vi "Filter StartRun Msg.vi"(10 "Current List":string, 11 "New RT Events":string) -> (3 "New List":string)   [LabVIEW 2015]
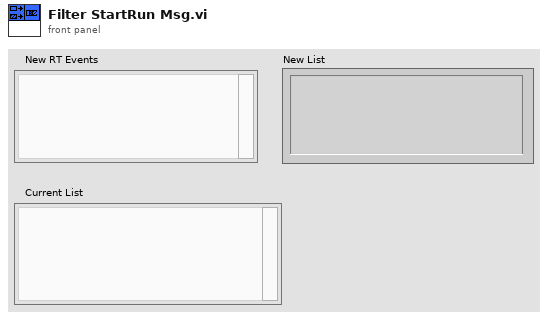
[diagram p1: front panel]
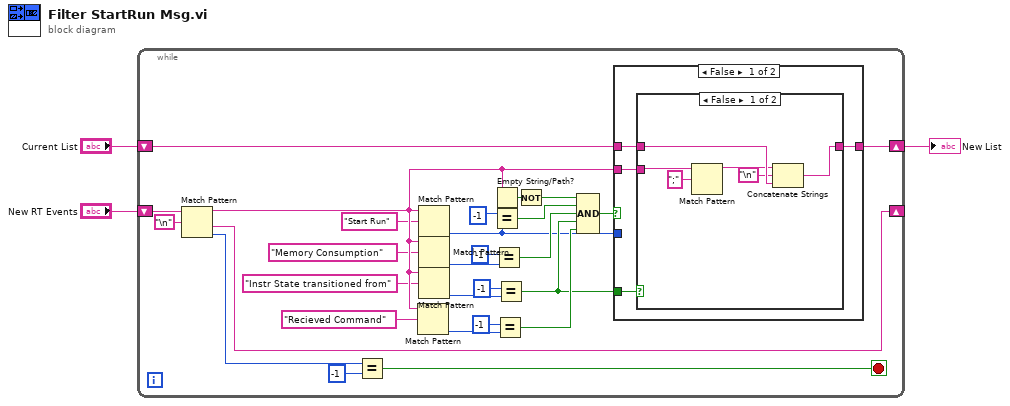
[diagram p0: block diagram]
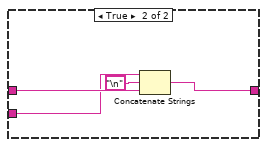
[diagram p3: hidden frame]
diagram:
  n1 = while {
    shift-right: [w5] -> _
    shift-left: "New RT Events" -> [w7]
    shift-right: [w4] -> w1
    shift-left: "Current List" -> [w8]
    stop <- w30 stop-if-true
    n2 = Match Pattern(string=w7, regular expression="\n") -> (before substring=w28:string, after substring=w5:string, offset past match=w6:i32)  [unwired: 1 in, 1 out]
    n3 = Equal?(x=w6, y=-1) -> (x = y?=w30:bool)
    n4 = Match Pattern(string=w28, regular expression="Recieved Command") -> (offset past match=w25:i32)  [unwired: 1 in, 3 out]
    n5 = Match Pattern(string=w28, regular expression="Start Run") -> (offset past match=w10:i32)  [unwired: 1 in, 3 out]
    n6 = Match Pattern(string=w28, regular expression="Memory Consumption") -> (offset past match=w13:i32)  [unwired: 1 in, 3 out]
    n7 = Match Pattern(string=w28, regular expression="Instr State transitioned from") -> (offset past match=w18:i32)  [unwired: 1 in, 3 out]
    n8 = Empty String/Path?(string/path=w28) -> (empty?=w11:bool)
    n9 = Equal?(x=-1 ("y"), y=w10) -> (x = y?=w20:bool)
    n10 = Equal?(x=-1 ("y"), y=w13) -> (x = y?=w21:bool)
    n11 = Equal?(x=-1 ("y"), y=w25) -> (x = y?=w29:bool)
    n12 = Equal?(x=-1 ("y"), y=w18) -> (x = y?=w23:bool)
    n13 = Not(x=w11) -> (.not. x?=w19:bool)
    n14 = Compound Arithmetic op=AND(w19, w20, w21, w23, w29) -> (w22:bool)
    n15 = case shown="False" w22 {
      tunnel: w8 -> [w35 w45]
      tunnel: w28 -> [w33 w44]
      tunnel: [w34 w46] -> w4
      tunnel: w10 -> [_ _]
      tunnel: w23 -> [w32 _]
      frame False {
        n16 = case shown="False" w32 {
          tunnel: w35 -> [w41 w42]
          tunnel: [w37 w42] -> w34
          tunnel: w33 -> [w40 _]
          frame False {
            n17 = Match Pattern(string=w40, regular expression=";") -> (before substring=w36:string)  [unwired: 1 in, 3 out]
            n18 = Concatenate Strings(w36, "\n", w41) -> (w37:string)
          }
          frame True {
          }
        }
      }
      frame True {
        n19 = Concatenate Strings(w44, "\n", w45) -> (w46:string)
      }
    }
  }
  "New List" <- w1
